vi "String to Vector.vi"(1 "Vector Dimension":i32, 2 "String Input":string) -> (0 "Vector":dbl[](array[numeric]))   [LabVIEW 2014]
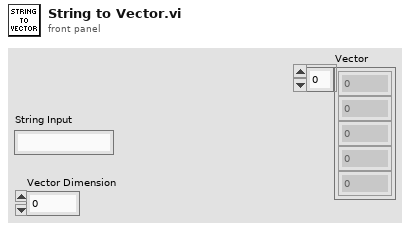
[diagram p1: front panel]
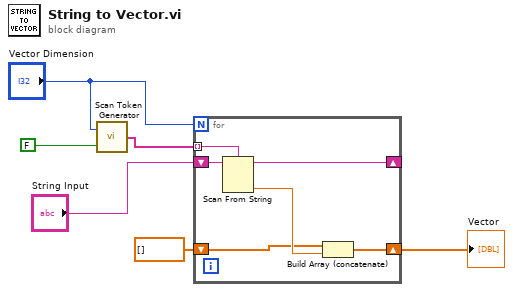
[diagram p0: block diagram]
diagram:
  n1 = call "Scan Token Generator.vi"("Matrix"=FALSE, "Martix Dimension"="Vector Dimension") -> ("Array"=w5:string[])
  n2 = for {
    N: "Vector Dimension" -> [_]
    tunnel: w5 -> [w10] mode=indexing
    shift-right: [w9] -> _
    shift-left: "String Input" -> [w12]
    shift-right: [w7] -> w2
    shift-left: dbl[] [] -> [w8]
    n3 = Scan From String(format string=w10, input string=w12) -> (remaining string=w9:string, output 1=w11:dbl)  [unwired: 3 in, 2 out]
    n4 = Build Array (concatenate)(w8, w11) -> (w7:dbl[])
  }
  "Vector" <- w2
